vi "thermo_declusterize_single_channel.vi"(0 "thermo channel":T1[](array[typedef])) -> (1 "temp":dbl[](array[numeric]), 2 "RH":dbl[](array[numeric]), 3 "pres":dbl[](array[numeric]))   [LabVIEW 2020]
uses:
  thermo_read.ctl
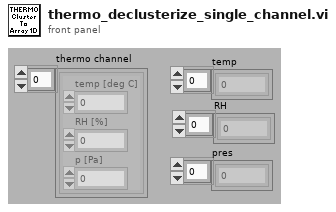
[diagram p1: front panel]
types:
  T1 = typedef "thermo_read.ctl" = cluster{"temp [deg C]":dbl, "RH [%]":dbl, "p [Pa]":dbl}
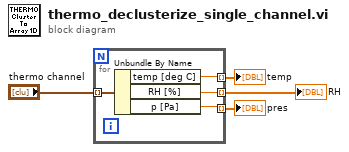
[diagram p0: block diagram]
diagram:
  n1 = for {
    tunnel: "thermo channel" -> [w8] mode=indexing
    tunnel: [w7] -> w4 mode=indexing
    tunnel: [w6] -> w3 mode=indexing
    tunnel: [w5] -> w2 mode=indexing
    n2 = Unbundle By Name(w8) -> ("temp [deg C]"=w7:dbl, "RH [%]"=w6:dbl, "p [Pa]"=w5:dbl)
  }
  "temp" <- w4
  "RH" <- w3
  "pres" <- w2
